vi "Execute PC Benchmarking.vi"   [LabVIEW 2014]
uses:
  <vilib>/Utility/error.llb/DialogType.ctl
  <vilib>/Wiresmith Technology/LabVIEW CLI/CLI Class/CLI.lvclass
types:
  T1 = typedef "DialogType.ctl" = u16
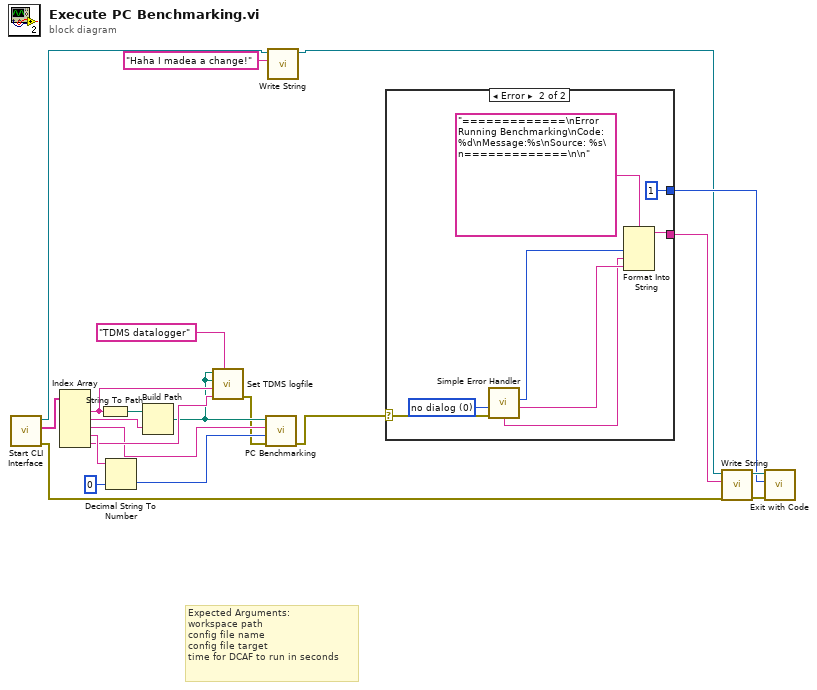
[diagram p0: block diagram]
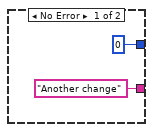
[diagram p2: hidden frame]
diagram:
  # "Expected Arguments:\nworkspace path\nconfig file name\nconfig file target\ntime for DCAF to run in seconds"
  n1 = call <vilib>:"Start CLI Interface.vi"() -> ("error out"=w14:errorcluster, "Custom Parameters"=w21:string[], "CLI out"=w3:refnum<class "CLI.lvclass">)  [unwired: 9 in]
  n2 = Index Array(array=w21) -> (element #1=w9:string, element #2=w19:string, element #3=w7:string, element #4=w13:string, element #5=w10:string)  [unwired: 5 in]
  n3 = String To Path(string=w9) -> (path=w20:path)
  n4 = Decimal String To Number(string=w13, default (0L)=u32 0 ("default (0 I32)")) -> (number=w6:u32)  [unwired: 1 in, 1 out]
  n5 = Build Path(base path=w20, name or relative path=w19) -> (appended path=w8:path)
  n6 = call "Set TDMS logfile.vi"("TDMS Module Alias"="TDMS datalogger", "log name"=w10, "Log Directory"=w9, "Config File Save Path"=w8, "Config File Path"=w8) -> ("error out"=w5:errorcluster)  [unwired: 6 in]
  n7 = call "PC Benchmarking.vi"("error in"=w5, "run time"=w6, "target alias"=w7, "configuration file path"=w8) -> ("error out"=w4:errorcluster)  [unwired: 7 in]
  n8 = call <vilib>:"Write String.vi"("Text to Write"="Haha I madea a change!", "CLI in"=w3) -> ("CLI out"=w2:refnum<class "CLI.lvclass">)  [unwired: 8 in, 1 out]
  n9 = case shown="Error" w4 {
    selector: w4 -> [_ w28]
    tunnel: ["Another change" w24] -> w16
    tunnel: [0 ("Exit Code (0)") 1 ("Exit Code (0)")] -> w15
    frame No Error {
    }
    frame Error {
      w29 = T1 0 items=["no dialog", "OK message", "continue or stop message", "OK message + warnings", "continue/stop + warnings"] ("type of dialog (OK msg:1)")
      n10 = call <vilib>:"Simple Error Handler.vi"("type of dialog (OK msg:1)"=w29, "error in (no error)"=w28) -> ("code out"=w27:i32, "source out"=w26:string, "message"=w25:string)  [unwired: 3 in, 2 out]
      n11 = Format Into String(format string="=============\nError Running Benchmarking\nCode: %d\nMessage:%s\nSource: %s\n=============\n\n", w27, w25, w26) -> (resulting string=w24:string)  [unwired: 2 in, 1 out]
    }
  }
  n12 = call <vilib>:"Write String.vi"("error in (no error)"=w14, "Text to Write"=w16, "CLI in"=w2) -> ("error out"=w18:errorcluster, "CLI out"=w17:refnum<class "CLI.lvclass">)  [unwired: 7 in]
  n13 = call <vilib>:"Exit with Code.vi"("error in (no error)"=w18, "Exit Code (0)"=w15, "CLI in"=w17) -> ()  [unwired: 8 in, 1 out]
